vi "XYStage.ReadPosition.vi"(8 "error in (no error)":errorcluster, 11 "XYStage.Simulated":refnum<class "XYStage.Simulated.lvclass">) -> (0 "error out":errorcluster, 1 "Counts out":T1, 2 "Position":T2, 3 "XYStage.Simulated out":refnum<class "XYStage.Simulated.lvclass">)   [LabVIEW 2015, in "XYStage.Simulated.lvclass"]
doc: "---------------------------------------------------------------\nJKI State Machine Objects™\nhttp://jki.net/state-machine-objects/\nCopyright (C) 2005-2015, JKI <info@jki.net>\nALL RIGHTS RESERVEDJKI State Machine Objects (SMO) 1.0.0.5\nJKI - JKI\nCopyright (c) 2016, JKI"
uses:
  XYStage.Simulated.lvclass
  XYStage/Typedefs/(real)Coords--Cluster.ctl
  XYStage/Typedefs/(counts)Coords--Cluster.ctl
  XYStage/XYStage.lvclass
panel:
  # "For instructions on how to use the JKI State Machine Objects, examples and video tutorials, visit:\nhttp://jki.net/state-machine-objects/\n\nJKI State Machine Objects™\nhttp://jki.net/state-machine-objects/\nCopyright (C) 2005-2015, JKI <info@jki.net>\nALL RIGHTS RESERVED"
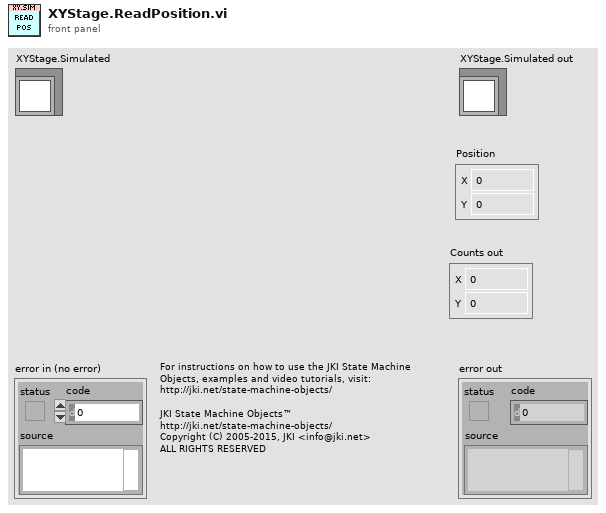
[diagram p1: front panel]
types:
  T1 = typedef "XYStage.lvclass/(counts)Coords--Cluster.ctl" = cluster{"X":i32, "Y":i32}
  T2 = typedef "XYStage.lvclass/(real)Coords--Cluster.ctl" = cluster{"X":dbl, "Y":dbl}
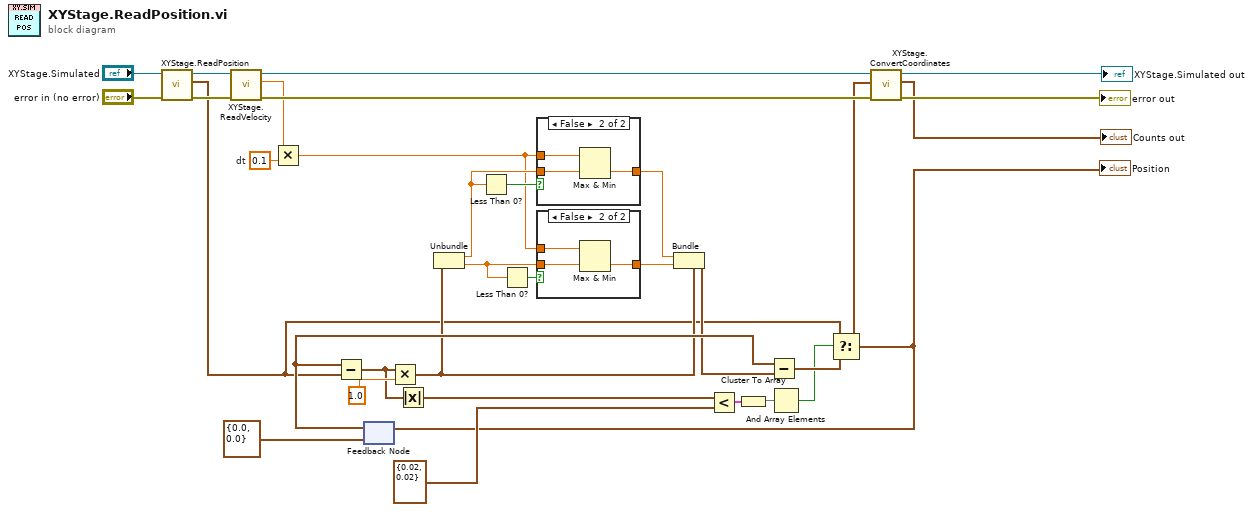
[diagram p0: block diagram]
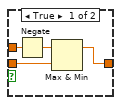
[diagram p2: hidden frame]
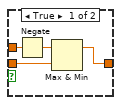
[diagram p3: hidden frame]
diagram:
  w19 = 0.1  # dt
  n1 = call-parent "XYStage.ReadPosition.vi"("error in (no error)"="error in (no error)", "XYStage"="XYStage.Simulated") -> ("error out"=w4:errorcluster, "Position"=w3:T2, "XYStage out"=w5:refnum<class "XYStage.Simulated.lvclass">)  [unwired: 6 in, 1 out]
  n2 = call-dynamic "XYStage.ReadVelocity.vi"("error in (no error)"=w4, "XYStage in"=w5) -> ("error out"=w21:errorcluster, "Velocity (units/s)"=w20:dbl, "XYStage out"=w22:refnum<class "XYStage.Simulated.lvclass">)  [unwired: 6 in, 1 out]
  n3 = Multiply(x=w20, y=w19) -> (x*y=w11:dbl)
  n4 = feedback #1(T2 {"X"=0.0, "Y"=0.0} ("Coords")) -> (w31:T2)
  n5 = Subtract(x=w31, y=w3) -> (x-y=w29:T2)
  n6 = Multiply(x=w29, y=1.0) -> (x*y=w18:T2)
  n7 = Absolute Value(x=w29) -> (abs(x)=w28:T2)
  n8 = Unbundle(w18) -> ("X"=w14:dbl, "Y"=w12:dbl)
  n9 = Less Than 0?(x=w14) -> (x < 0?=w16:bool)
  n10 = Less Than 0?(x=w12) -> (x < 0?=w13:bool)
  n11 = case shown="False" w16 {
    tunnel: w11 -> [w36 w39]
    tunnel: w14 -> [w35 w38]
    tunnel: [w34 w37] -> w15
    frame True {
      n12 = Negate(x=w36) -> (-x=w33:dbl)
      n13 = Max & Min(x=w33, y=w35) -> (max(x,y)=w34:dbl)  [unwired: 1 out]
    }
    frame False {
      n14 = Max & Min(x=w39, y=w38) -> (min(x,y)=w37:dbl)  [unwired: 1 out]
    }
  }
  n15 = case shown="False" w13 {
    tunnel: w11 -> [w43 w46]
    tunnel: w12 -> [w42 w45]
    tunnel: [w41 w44] -> w10
    frame True {
      n16 = Negate(x=w43) -> (-x=w40:dbl)
      n17 = Max & Min(x=w40, y=w42) -> (max(x,y)=w41:dbl)  [unwired: 1 out]
    }
    frame False {
      n18 = Max & Min(x=w46, y=w45) -> (min(x,y)=w44:dbl)  [unwired: 1 out]
    }
  }
  n19 = Bundle(cluster=w18, "X"=w15, "Y"=w10) -> (w17:T2)
  n20 = Less?(x=w28, y=T2 {"X"=0.02, "Y"=0.02}) -> (x < y?=w25:cluster{"X":bool, "Y":bool})
  n21 = Cluster To Array(cluster=w25) -> (array=w24:bool[])
  n22 = Subtract(x=w31, y=w17) -> (x-y=w27:T2)
  n23 = And Array Elements(Boolean array=w24) -> (logical AND=w23:bool)
  n24 = Select(t=w3, s=w23, f=w27) -> (s? t:f=w1:T2)
  "Position" <- w1
  n25 = feedback-in #1(w1) -> ()
  n26 = call-dynamic "XYStage.ConvertCoordinates.vi"("error in (no error)"=w21, "Real Units Coords"=w1, "XYStage in"=w22) -> ("error out"=→"error out":errorcluster, "Counts out"=→"Counts out":T1, "XYStage out"=→"XYStage.Simulated out":refnum<class "XYStage.Simulated.lvclass">)  [unwired: 5 in, 1 out]
